vi "Modulate FPGA.vi"(0 "Action":T5, 3 "Dt":sgl=1.0, 7 "FPGA Output":T1, 9 "f0_set":T3 {"fl 5" format="%#.3g"; "f 4" format="%#.3g"; "f 3" format="%#.3g"; "f 1" format="%#.3g"; "f 2" format="%#.3g"}, 11 "error in":errorcluster) -> (4 "Drive":bool, 15 "error out":errorcluster)   [LabVIEW 2012]
doc: "<B>Change FPGA State</B> is called when a change the PAS high frequency signals is desired."
uses:
  <vilib>/rvi/interface/nirviReadWriteControl/nirviReadWriteControl.xnode
  <vilib>/userdefined/High Color/nirio_resource_hc.ctl
  <vilib>/rvi/interface/nirviOpenFPGA/nirviOpenFPGA.xnode
  <vilib>/rvi/interface/nirviCloseFPGA/nirviCloseFPGA.xnode
  Utilities/FPGA/Controls/FPGA Signal.ctl
  PAS/Controls/FPGA/FPGA FG Action.ctl
  FPGA Bitfiles/CRDS_PAS.lvproj_FPGA Target_FPGA IO.vi.lvbitx
  NiFpgaLv.dll
  <vilib>/Utility/error.llb/Error Cluster From Error Code.vi
  <vilib>/rvi/errors/niLvFpgaAdjustHostInterfaceError.vi
  <vilib>/FPGAPlugInAG/PXI-7841R/niLvFpga_Close_PXI-7841R.vi
  <vilib>/FPGAPlugInAG/PXI-7841R/niLvFpga_Open_PXI-7841R.vi
  Reusable/PAS/Main/Controls/Laser Modulation.ctl
  Utilities/FPGA/Controls/FPGAConfig.ctl
panel:
  out "current time":timestamp
  out "Stopped":bool
  out "SquareOut":T4
  out "OtherOut":T4
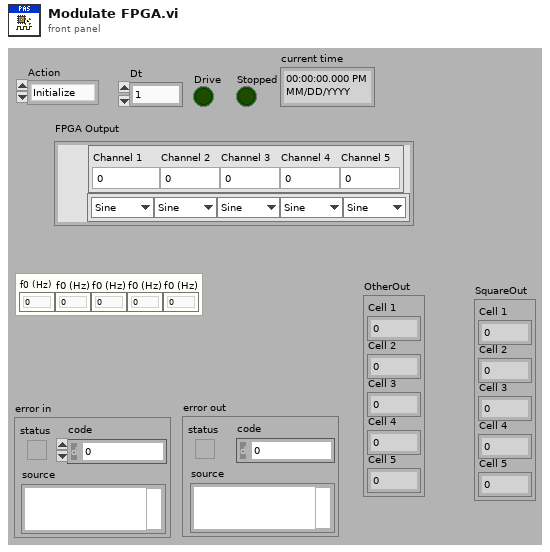
[diagram p1: front panel]
types:
  T1 = typedef "FPGAConfig.ctl" = cluster{"Span":cluster{"ch 1":sgl, "ch 2":sgl, "ch 3":sgl, "ch 4":sgl, "ch 5":sgl}, "mod":cluster{"ch 1":T2, "ch 2":T2, "ch 3":T2, "ch 4":T2, "ch 5":T2}}
  T2 = typedef "Laser Modulation.ctl" = enum8{"Sine", "Square"}
  T3 = cluster{"f 1":sgl, "f 2":sgl, "f 3":sgl, "f 4":sgl, "fl 5":sgl}
  T4 = cluster{"Cell 1":i16, "Cell 2":i16, "Cell 3":i16, "Cell 4":i16, "Cell 5":i16}
  T5 = typedef "FPGA FG Action.ctl" = enum8{"Initialize", "Laser", "Speaker", "Change Drive", "Check Drive", "Off", "Stop"}
  T6 = typedef "nirio_resource_hc.ctl" = tag
  T7 = typedef "FPGA Signal.ctl" = enum16{"Laser", "None", "Speaker"}
  T8 = cluster{"ch 1":sgl, "ch 2":sgl, "ch 3":sgl, "ch 4":sgl, "ch 5":sgl}
  T9 = cluster{"ch 1":T2, "ch 2":T2, "ch 3":T2, "ch 4":T2, "ch 5":T2}
  T10 = typedef "FxdPt Props.ctl" = cluster{"f0":fxp<+,32,0>, "Scale":fxp<+,14,1>, "Offset":i16, "Mod":T2}
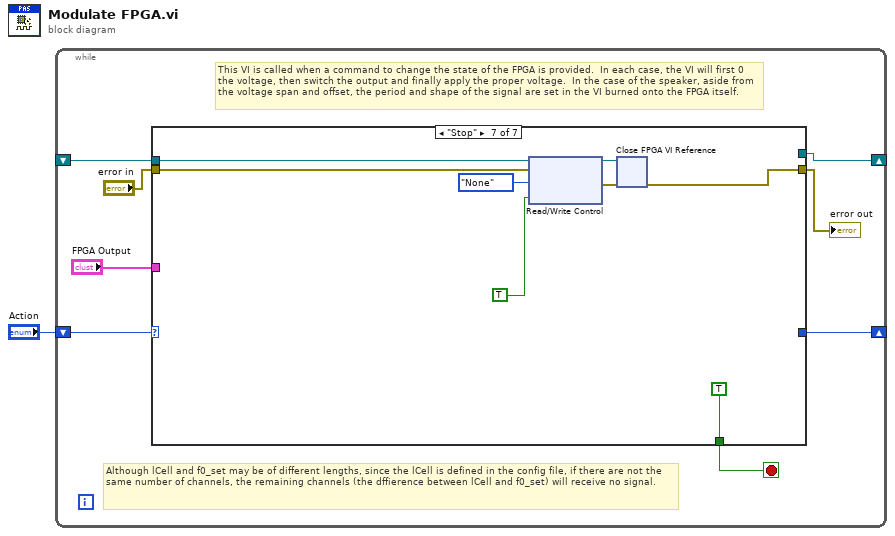
[diagram p0: block diagram]
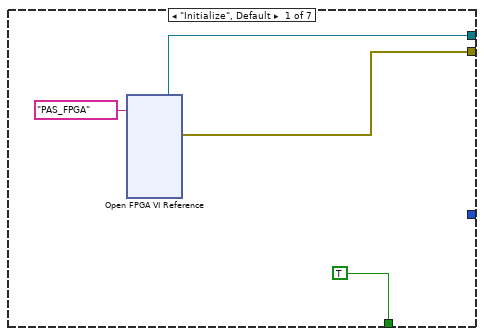
[diagram p2: hidden frame]
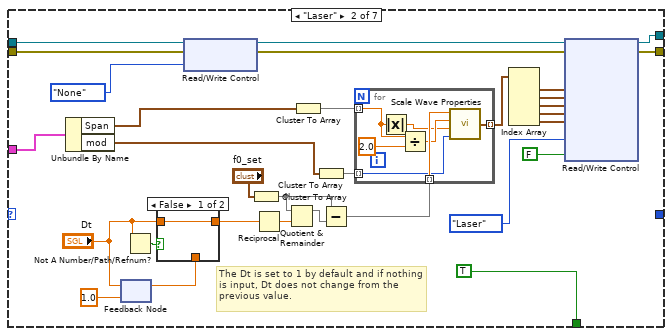
[diagram p3: hidden frame]
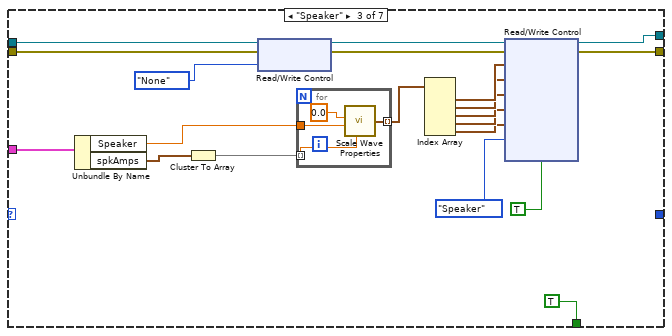
[diagram p5: hidden frame]
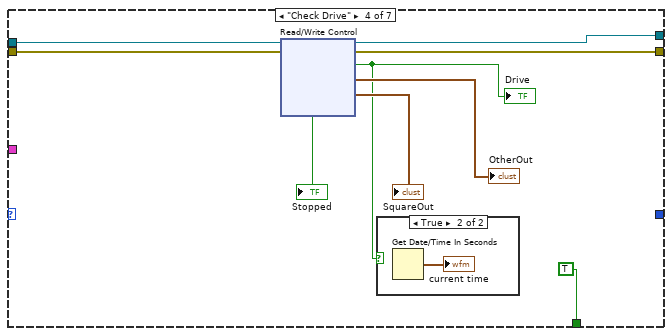
[diagram p6: hidden frame]
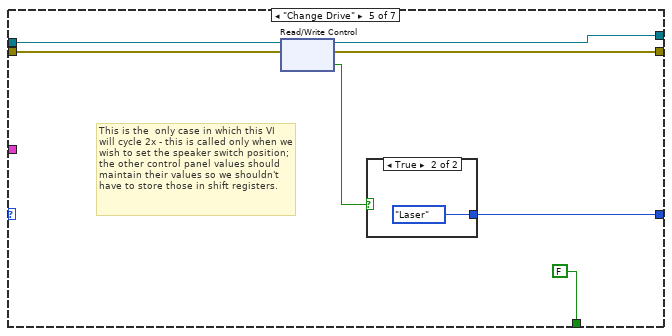
[diagram p8: hidden frame]
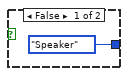
[diagram p9: hidden frame]
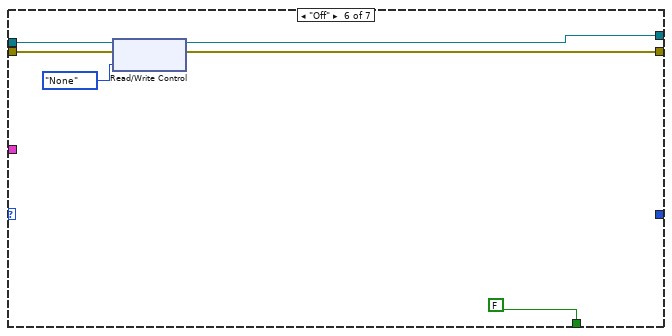
[diagram p10: hidden frame]
diagram:
  n1 = while {
    shift-right: [w2] -> _
    shift-left: _ -> [w7]
    shift-right: [w4] -> _
    shift-left: "Action" -> [w5]
    stop <- w6 stop-if-true
    # "Although lCell and f0_set may be of different lengths, since the lCell is defined in the config file, if there are not the same number of channels, the remaining channels (the dffierence between lCell and f0_set) will receive no signal."
    # "This VI is called when a command to change the state of the FPGA is provided.  In each case, the VI will first 0 the voltage, then switch the output and finally apply the proper voltage.  In the case of the speaker, aside from the voltage span and offset, the period and shape of the signal are set in the VI burned onto the FPGA itself."
    n2 = case shown="\"Stop\"" w5 {
      tunnel: "error in" -> [_ w34 w72 w85 w92 w101 w107]
      tunnel: [w12 w44 w73 w84 w89 w100 w108] -> w9
      tunnel: w7 -> [_ w32 w70 w86 w93 w102 w105]
      tunnel: "FPGA Output" -> [_ w22 w68 _ _ _ _]
      tunnel: [TRUE TRUE TRUE TRUE FALSE FALSE TRUE] -> w6
      tunnel: [_ _ _ _ w90 _ _] -> w4
      tunnel: [w10 w14 w54 w78 w88 w97 _] -> w2
      frame "Initialize", Default {
        n3 = xnode "Open FPGA VI Reference"("resource name"=T6 "PAS_FPGA") -> ("FPGA VI Reference Out"=w10:refnum<k20>, "error out"=w12:errorcluster)  [unwired: 1 in]
      }
      frame "Laser" {
        # "The Dt is set to 1 by default and if nothing is input, Dt does not change from the previous value."
        n4 = Unbundle By Name(w22) -> ("Span"=w15:T8, "mod"=w24:T9)
        n5 = feedback-in #1("Dt") -> ()
        n6 = feedback #1(sgl 1.0 ("Dt")) -> (w35:sgl)
        n7 = Not A Number/Path/Refnum?(number/path/refnum="Dt") -> (NaN/Path/Refnum?=w37:bool)
        n8 = case shown="False" w37 {
          tunnel: "Dt" -> [w45 _]
          tunnel: [w45 w46] -> w25
          tunnel: w35 -> [_ w46]
          frame False {
          }
          frame True {
          }
        }
        n9 = xnode "Read/Write Control"("FPGA VI Reference In"=w32, "error in"=w34, "WaveType"=FPGA_Signal."None") -> ("FPGA VI Reference Out"=w31:refnum<k20>, "error out"=w33:errorcluster)
        n10 = Cluster To Array(cluster="f0_set") -> (array=w28:sgl[])
        n11 = Reciprocal(x=w25) -> (1/x=w30:sgl)
        n12 = Quotient & Remainder(x=w28, y=w30) -> (x-y*floor(x/y)=w29:sgl[])  [unwired: 1 out]
        n13 = Cluster To Array(cluster=w15) -> (array=w17:sgl[])
        n14 = Cluster To Array(cluster=w24) -> (array=w23:T2[])
        n15 = Subtract(x=w28, y=w29) -> (x-y=w27:sgl[])
        n16 = for {
          tunnel: [w53] -> w43 mode=indexing
          tunnel: w27 -> [w52] mode=indexing
          tunnel: w23 -> [w48] mode=indexing
          tunnel: w17 -> [w47] mode=indexing
          n17 = Absolute Value(x=w47) -> (abs(x)=w49:sgl)
          n18 = Divide(x=w47, y=sgl 2.0) -> (x/y=w50:sgl)
          n19 = call "Scale Wave Properties.vi"("f0"=w52, "DCoffset"=w50, "Vspan"=w49, "Mod"=w48) -> ("FXP Props"=w53:T10)  [unwired: 1 in]
        }
        n20 = Index Array(array=w43) -> (element #1=w42:T10, element #2=w41:T10, element #3=w40:T10, element #4=w39:T10, element #5=w38:T10)  [unwired: 5 in]
        n21 = xnode "Read/Write Control"("FPGA VI Reference In"=w31, "error in"=w33, "Cell 1"=w42, "Cell 2"=w41, "Cell 3"=w40, "Cell 4"=w39, "Cell 5"=w38, "WaveType"=FPGA_Signal."Laser", "Drive"=FALSE) -> ("FPGA VI Reference Out"=w14:refnum<k20>, "error out"=w44:errorcluster)
      }
      frame "Speaker" {
        n22 = Unbundle By Name(w68) -> ("Speaker"=w55:sgl, "spkAmps"=w66:T8)
        n23 = Cluster To Array(cluster=w66) -> (array=w67:sgl[])
        n24 = xnode "Read/Write Control"("FPGA VI Reference In"=w70, "error in"=w72, "WaveType"=FPGA_Signal."None") -> ("FPGA VI Reference Out"=w69:refnum<k20>, "error out"=w71:errorcluster)
        n25 = for {
          tunnel: w55 -> [w77]
          tunnel: [w76] -> w65 mode=indexing
          tunnel: w67 -> [w74] mode=indexing
          n26 = call "Scale Wave Properties.vi"("DCoffset"=sgl 0.0, "Vspan"=w77, 4:w74) -> ("FXP Props"=w76:T10)  [unwired: 2 in]
        }
        n27 = Index Array(array=w65) -> (element #1=w64:T10, element #2=w63:T10, element #3=w62:T10, element #4=w61:T10, element #5=w60:T10)  [unwired: 5 in]
        n28 = xnode "Read/Write Control"("FPGA VI Reference In"=w69, "error in"=w71, "Cell 1"=w64, "Cell 2"=w63, "Cell 3"=w62, "Cell 4"=w61, "Cell 5"=w60, "WaveType"=FPGA_Signal."Speaker", "Drive"=TRUE) -> ("FPGA VI Reference Out"=w54:refnum<k20>, "error out"=w73:errorcluster)
      }
      frame "Check Drive" {
        n29 = xnode "Read/Write Control"("FPGA VI Reference In"=w86, "error in"=w85) -> ("FPGA VI Reference Out"=w78:refnum<k20>, "error out"=w84:errorcluster, "Drive"=w79:bool, "OtherOut"=→"OtherOut":T4, "SquareOut"=→"SquareOut":T4, "Stopped"=→"Stopped":bool)
        "Drive" <- w79
        n30 = case shown="True" w79 {
          frame False {
          }
          frame True {
            n31 = Get Date/Time In Seconds() -> (seconds since 1Jan1904=→"current time":timestamp)
          }
        }
      }
      frame "Change Drive" {
        # "This is the  only case in which this VI will cycle 2x - this is called only when we wish to set the speaker switch position; the other control panel values should maintain their values so we shouldn't have to store those in shift registers."
        n32 = xnode "Read/Write Control"("FPGA VI Reference In"=w93, "error in"=w92) -> ("FPGA VI Reference Out"=w88:refnum<k20>, "error out"=w89:errorcluster, "Drive"=w91:bool)
        n33 = case shown="True" w91 {
          tunnel: [FPGA_FG_Action."Speaker" ("Action") FPGA_FG_Action."Laser" ("Action")] -> w90
          frame False {
          }
          frame True {
          }
        }
      }
      frame "Off" {
        n34 = xnode "Read/Write Control"("FPGA VI Reference In"=w102, "error in"=w101, "WaveType"=FPGA_Signal."None") -> ("FPGA VI Reference Out"=w97:refnum<k20>, "error out"=w100:errorcluster)
      }
      frame "Stop" {
        n35 = xnode "Read/Write Control"("FPGA VI Reference In"=w105, "error in"=w107, "WaveType"=FPGA_Signal."None", "stop"=TRUE) -> ("FPGA VI Reference Out"=w106:refnum<k20>, "error out"=w110:errorcluster)
        n36 = xnode "Close FPGA VI Reference"("FPGA VI Reference In"=w106, "error in"=w110) -> ("error out"=w108:errorcluster)
      }
    }
    "error out" <- w9
  }
